vi "Write Style.vi"(8 "error in (no error)":errorcluster, 9 "Style String":string, 10 "Style index (-1)":i32=-1, 11 "Control in":refnum<class "Control.lvclass">) -> (0 "error out":errorcluster, 3 "Control out":refnum<class "Control.lvclass">)   [LabVIEW 2012, in "Control.lvclass"]
doc: "Accessor VI for the control class"
uses:
  Control.lvclass
  Control.lvclass/Control.ctl
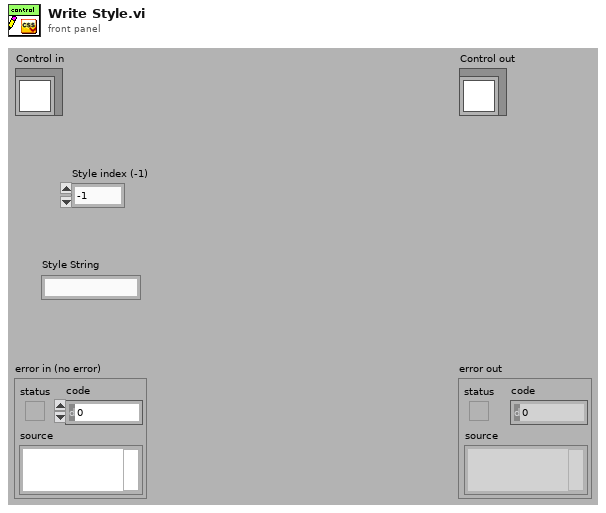
[diagram p1: front panel]
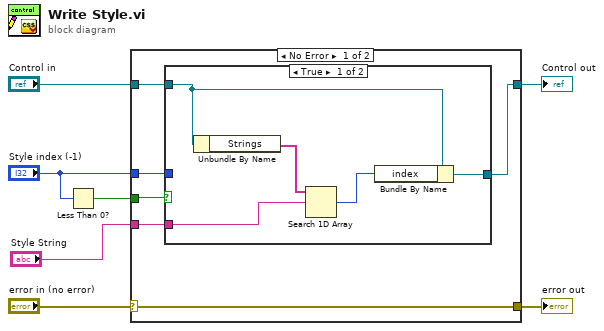
[diagram p0: block diagram]
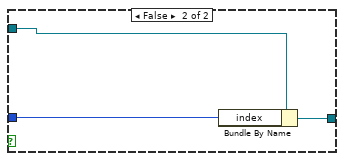
[diagram p2: hidden frame]
diagram:
  n1 = Less Than 0?(x="Style index (-1)") -> (x < 0?=w2:bool)
  n2 = case shown="No Error" "error in (no error)" {
    selector: "error in (no error)" -> [w13 w22]
    tunnel: [w13 w22] -> w6
    tunnel: [w12 w23] -> w4
    tunnel: "Control in" -> [w10 w23]
    tunnel: "Style index (-1)" -> [w11 _]
    tunnel: w2 -> [w9 _]
    tunnel: "Style String" -> [w8 _]
    frame No Error {
      n3 = case shown="True" w9 {
        tunnel: [w18 w21] -> w12
        tunnel: w11 -> [_ w20]
        tunnel: w10 -> [w17 w19]
        tunnel: w8 -> [w15 _]
        frame True {
          n4 = Unbundle By Name(w17) -> ("Strings"=w16:string[])
          n5 = Search 1D Array(1D array=w16, element=w15) -> (index of element=w14:i32)  [unwired: 1 out]
          n6 = Bundle By Name(cluster=w17, "index"=w14) -> (w18:refnum<class "Control.lvclass">)
        }
        frame False {
          n7 = Bundle By Name(cluster=w19, "index"=w20) -> (w21:refnum<class "Control.lvclass">)
        }
      }
    }
    frame Error {
    }
  }
  "error out" <- w6
  "Control out" <- w4
